vi "Load ROI from File.vi"(8 "error in (no error)":errorcluster, 10 "Report File":path, 11 "IMAQ Display in":refnum<class "HIJ Vision Display.lvclass">) -> (0 "error out":errorcluster, 3 "IMAQ Display out":refnum<class "HIJ Vision Display.lvclass">)   [LabVIEW 2014, in "HIJ Vision Display.lvlib" / "HIJ Vision Display.lvclass"]
uses:
  HIJ Vision Display.lvclass
  HIJ Vision Display.lvclass/HIJ Vision Display.ctl
  <vilib>/Utility/config.llb/NI_LVConfig.lvlib
  Utility/POLARIS Vision utility.lvlib
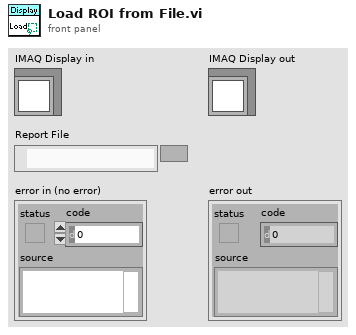
[diagram p1: front panel]
types:
  T1 = typedef "NI_LVConfig.lvlib/Config Data RefNum.ctl" = refnum<k1>
  T2 = typedef "ROI Descriptor" = cluster{"Global Rectangle":i32[], "Contours":cluster{"ID":enum32{"External", "Internal"}, "Type":u32, "Coordinates":i32[]}[]}
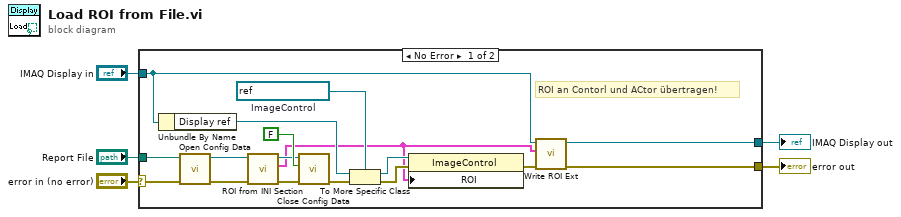
[diagram p0: block diagram]
diagram:
  n1 = case shown="No Error" "error in (no error)" {
    selector: "error in (no error)" -> [w17 w24]
    tunnel: [w14 w24] -> w4
    tunnel: [w15 w23] -> w2
    tunnel: "IMAQ Display in" -> [w13 w23]
    tunnel: "Report File" -> [w18 _]
    frame No Error {
      w11 = refnum<vi> refnum  # ImageControl
      # "ROI an Contorl und ACtor übertragen!"
      n2 = Unbundle By Name(w13) -> ("Display ref"=w12:refnum<vi>)
      n3 = call <vilib>:"Open Config Data.vi"("error in (no error)"=w17, "configuration file path"=w18) -> ("error out"=w20:errorcluster, "refnum"=w21:T1)  [unwired: 7 in, 1 out]
      n4 = call "ROI from INI Section.vi"("error in (no error)"=w20, "refnum in"=w21) -> ("error out"=w16:errorcluster, "ROI"=w8:T2, "refnum out"=w19:T1)  [unwired: 7 in]
      n5 = call <vilib>:"Close Config Data.vi"("error in (no error)"=w16, "write file if changed (T)"=FALSE, "refnum"=w19) -> ("error out"=w7:errorcluster)  [unwired: 7 in, 1 out]
      n6 = To More Specific Class(target class=w11, reference=w12, error in=w7) -> (specific class reference=w10:refnum<vi>, error out=w9:errorcluster)
      n7 = property class="ImageControl"(reference=w10, error in=w9, "ROI"=w8) -> (error out=w6:errorcluster)  [unwired: 1 out]
      n8 = call "Write ROI Ext.vi"("error in (no error)"=w6, "ROI Descriptor"=w8, "IMAQ Display in"=w13) -> ("error out"=w14:errorcluster, "IMAQ Display out"=w15:refnum<class "HIJ Vision Display.lvclass">)  [unwired: 7 in]
    }
    frame Error {
    }
  }
  "error out" <- w4
  "IMAQ Display out" <- w2
